vi "Actor Core.vi"(8 "error in":errorcluster, 11 "Power Supply in":refnum<class "Power Supply.lvclass">) -> (0 "error out":errorcluster, 3 "Actor out":refnum<class "Actor.lvclass">)   [LabVIEW 2020, in "Power Supply.lvlib" / "Power Supply.lvclass"]
doc: "(<B>Filename</B>: Actor Framework.lvlib:Actor.lvclass:Actor Core.vi)\n\nReceives messages to the actor, reacts to them, and initiates any error handling that may shut the actor down.\n\nDescendant classes may override this VI to append parallel tasks for the actor to complete while it handles messages. Overrides use the Call Parent Class Method node."
uses:
  Power Supply.lvclass
  C:/Program Files (x86)/National Instruments/LabVIEW 2020/vi.lib/ActorFramework/Actor/Actor.lvclass
  <vilib>/ActorFramework/Actor/Actor.lvclass
  <vilib>/ActorFramework/Actor/Actor.lvclass/Actor.ctl
  <vilib>/ActorFramework/Message Enqueuer/Message Enqueuer.lvclass/Message Enqueuer.ctl
  Power Supply.lvclass/Power Supply.ctl
  Power Supply Messages/Setup Msg/Setup Msg.lvclass/Setup Msg.ctl
  Power Supply Messages/Enable Disable Outuput Msg/Enable Disable Outuput Msg.lvclass/Enable Disable Outuput Msg.ctl
  <vilib>/ActorFramework/Message Enqueuer/Init from Existing Queue.vi
  <vilib>/ActorFramework/Message Enqueuer/Enqueue.vi
  Power Supply Messages/Setup Msg/Setup Msg.lvclass
  C:/Program Files (x86)/National Instruments/LabVIEW 2020/vi.lib/ActorFramework/Message/Message.lvclass
  Power Supply Messages/Enable Disable Outuput Msg/Enable Disable Outuput Msg.lvclass
  <vilib>/ActorFramework/Stop Msg/Stop Msg.lvclass
  <vilib>/ActorFramework/Message Priority Queue/Priority Enqueue.vi
  <vilib>/ActorFramework/Message Enqueuer/Message Enqueuer.lvclass
panel:
  out "Status":string
  in  "Output Status":bool
  in  "Setup":bool
  out "Output Status":bool
  in  "Amps":dbl
  in  "Volts":dbl
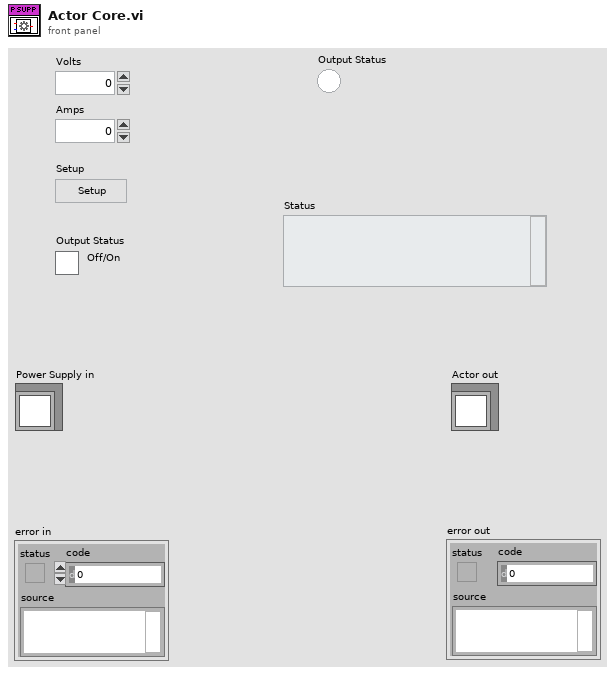
[diagram p1: front panel]
types:
  T1 = cluster{"Output Status":refnum<user-event>, "Stop":refnum<user-event>, "Status":refnum<user-event>}
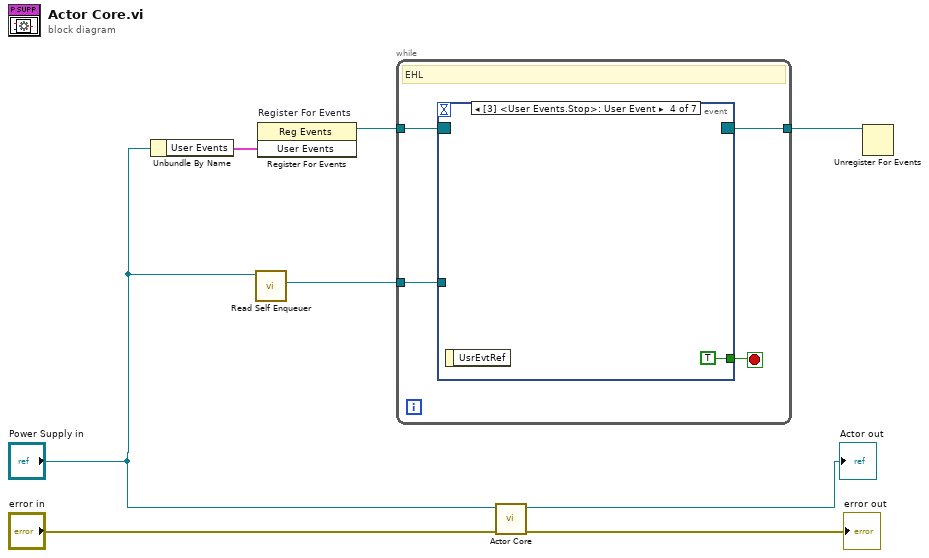
[diagram p0: block diagram]
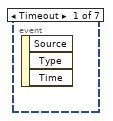
[diagram p2: hidden frame]
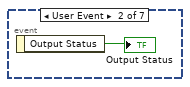
[diagram p3: hidden frame]
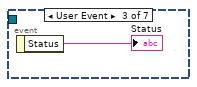
[diagram p4: hidden frame]
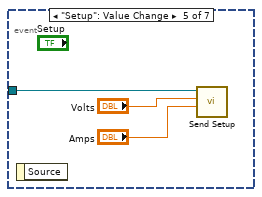
[diagram p5: hidden frame]
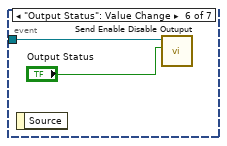
[diagram p6: hidden frame]
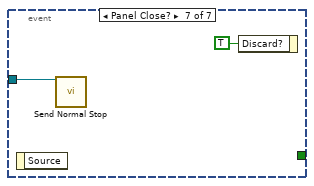
[diagram p7: hidden frame]
diagram:
  n1 = Unbundle By Name("Power Supply in") -> ("User Events"=w2:T1)
  n2 = call <vilib>:"Read Self Enqueuer.vi"("Actor"="Power Supply in") -> ("Self Enqueuer"=w3:refnum<class "Message Enqueuer.lvclass">)  [unwired: 10 in]
  n3 = register-events "Register For Events"(w2) -> (reference out=w5:refnum<event-registration>)  [unwired: 2 in, 1 out]
  n4 = while {
    tunnel: w5 -> [w12]
    tunnel: [w11] -> w4
    tunnel: w3 -> [w10]
    stop <- w9 stop-if-true
    # "EHL"
    n5 = event shown="[3] <User Events.Stop>: User Event" {
      selector: w12 -> [_ _ _ _ _ _ _]
      dyn-events: [_ _ _ _ _ _ _] -> w11
      timeout: _ -> [_ _ _ _ _ _ _]
      tunnel: w10 -> [_ _ _ _ w18 w20 w21]
      tunnel: [_ _ _ TRUE _ _ _] -> w9
      event Timeout {
        n6 = event-data() -> ()  [unwired: 1 in, 3 out]
      }
      event User Event {
        n7 = event-data() -> ("Output Status"=→"Output Status":bool)  [unwired: 1 in]
      }
      event User Event {
        n8 = event-data() -> ("Status"=→"Status":string)  [unwired: 1 in]
      }
      event User Event {
        n9 = event-data() -> ()  [unwired: 1 in, 1 out]
      }
      event "Setup": Value Change {
        n10 = event-data() -> ()  [unwired: 1 in, 1 out]
        n11 = call "Send Setup.vi"("Amps"="Amps", "Volts"="Volts", "Message Enqueuer"=w18) -> ()  [unwired: 7 in, 2 out]
      }
      event "Output Status": Value Change {
        n12 = event-data() -> ()  [unwired: 1 in, 1 out]
        n13 = call "Send Enable Disable Outuput.vi"("Enable/Disable"="Output Status", "Message Enqueuer"=w20) -> ()  [unwired: 8 in, 2 out]
      }
      event Panel Close? {
        n14 = event-data() -> ()  [unwired: 1 in, 1 out]
        n15 = call <vilib>:"Send Normal Stop.vi"("Message Enqueuer"=w21) -> ()  [unwired: 10 in, 1 out]
        n16 = event-data("Discard?"=TRUE) -> ()  [unwired: 1 in, 1 out]
      }
    }
  }
  n17 = call-parent "Actor Core.vi"("error in"="error in", "Actor in"="Power Supply in") -> ("error out"=→"error out":errorcluster, "Actor out"=→"Actor out":refnum<class "Actor.lvclass">)  [unwired: 8 in]
  n18 = Unregister For Events(event registration refnum=w4) -> ()  [unwired: 1 in, 1 out]
